vi "Move Error to Structure for Reporting.vi"(8 "error in (expected)":errorcluster, 10 "ESC Internal Data Structure (with types)":T2={"Test_File"=path "", "Status"="Done", "RF_Center_Freq"=0.0, "RF_Gain"=0.0, "BB_Gain"=0.0, "Error 2"="", "file_max"=0, "file_index"=0}, 11 "ESC Internal Data Structure (with strings)":T1={"Test_File"="", "Status"="Done", "RF_Center_Freq"="0", "RF_Gain"="0", "BB_Gain"="0", "Error"="", "file_max"="0", "file_index"="0"}) -> (0 "error out":errorcluster, 2 "ESC Internal Data Structure (with types) out":T2={"Test_File"=path "", "Status"="Done", "RF_Center_Freq"=0.0, "RF_Gain"=0.0, "BB_Gain"=0.0, "Error 2"="", "file_max"=0, "file_index"=0}, 3 "ESC Internal Data Structure (with strings) out":T1={"Test_File"="", "Status"="Done", "RF_Center_Freq"="0", "RF_Gain"="0", "BB_Gain"="0", "Error"="", "file_max"="0", "file_index"="0"})   [LabVIEW 2017]
uses:
  TypeDef/RF Internal Data Structure (string).ctl
  TypeDef/RF Internal Data Structure (types).ctl
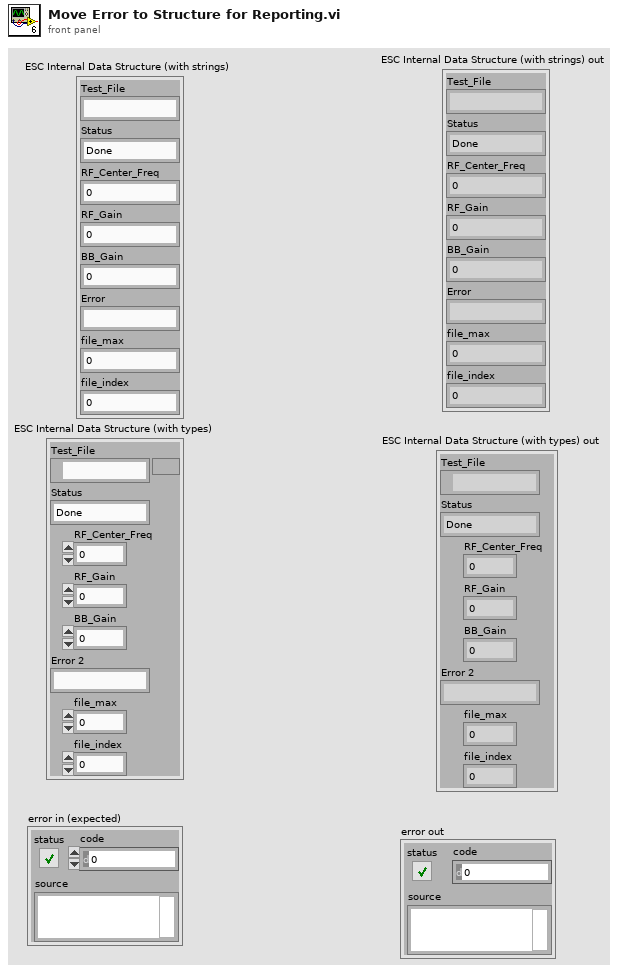
[diagram p1: front panel]
types:
  T1 = typedef "RF Internal Data Structure (string).ctl" = cluster{"Test_File":string, "Status":string, "RF_Center_Freq":string, "RF_Gain":string, "BB_Gain":string, "Error":string, "file_max":string, "file_index":string}
  T2 = typedef "RF Internal Data Structure (types).ctl" = cluster{"Test_File":path, "Status":string, "RF_Center_Freq":dbl, "RF_Gain":dbl, "BB_Gain":dbl, "Error 2":string, "file_max":u64, "file_index":u64}
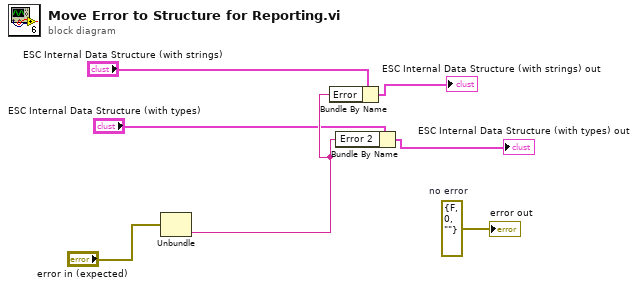
[diagram p0: block diagram]
diagram:
  w6 = errorcluster {"status"=FALSE, "code"=0, "source"=""}  # no error
  n1 = Unbundle("error in (expected)") -> ("source"=w5:string)  [unwired: 2 out]
  n2 = Bundle By Name(cluster="ESC Internal Data Structure (with strings)", "Error"=w5) -> (→"ESC Internal Data Structure (with strings) out":T1)
  n3 = Bundle By Name(cluster="ESC Internal Data Structure (with types)", "Error 2"=w5) -> (→"ESC Internal Data Structure (with types) out":T2)
  "error out" <- w6
